vi "ml_K Means_Update Means.vi"(8 "# of classes":i32=1, 9 "labels":i32[](array[numeric]), 11 "Samples":dbl[][](array[numeric])) -> (0 "# samples in classes":i32[](array[numeric]), 1 "labels dup":i32[](array[numeric]), 2 "Means":dbl[][](array[numeric]), 3 "Samples dup":dbl[][](array[numeric]))   [LabVIEW 2013, in "NILabs_MLT.lvlib"]
uses:
  <vilib>/addons/Machine Learning/NILabs_MLT.lvlib
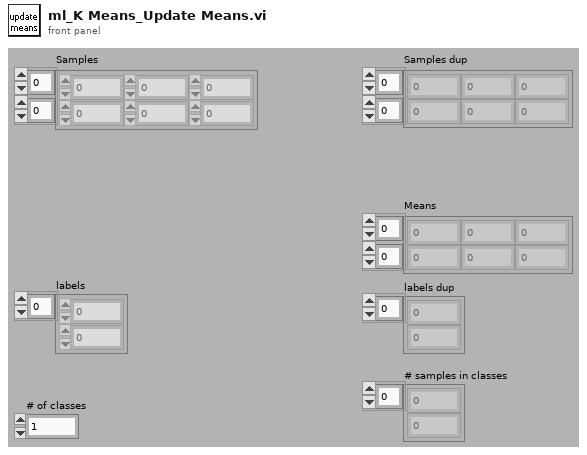
[diagram p1: front panel]
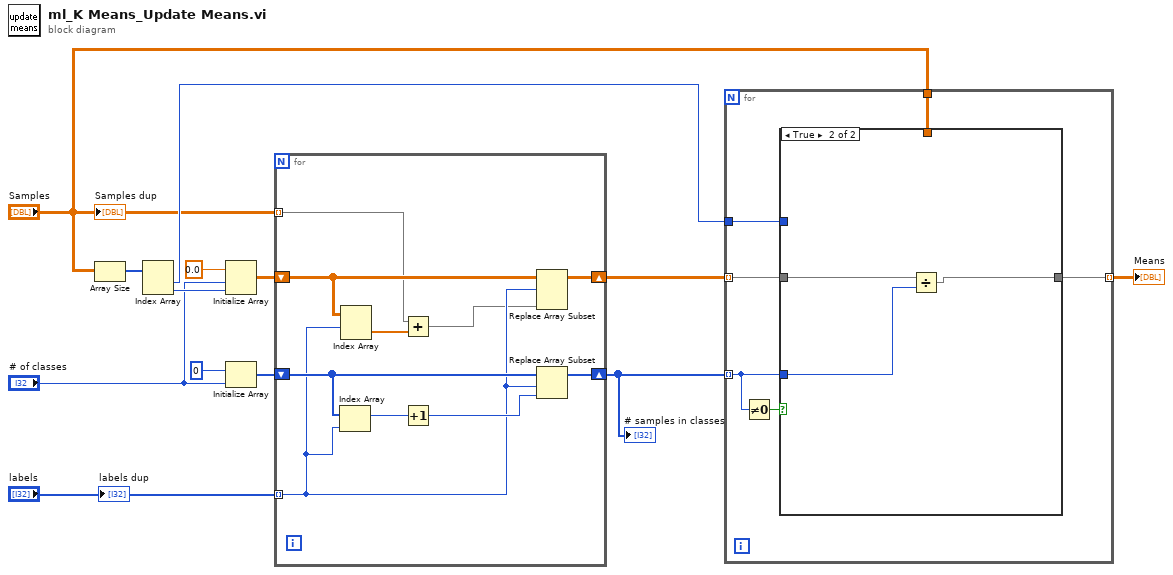
[diagram p0: block diagram]
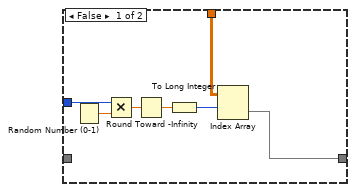
[diagram p2: hidden frame]
diagram:
  n1 = Array Size(array="Samples") -> (size(s)=w13:i32[])
  n2 = Index Array(array=w13) -> (element #1=w5:i32, element #2=w8:i32)  [unwired: 2 in]
  n3 = Initialize Array(0.0 ("element"), "# of classes", w8) -> (w9:dbl[][])
  n4 = Initialize Array(0 ("element"), "# of classes") -> (w10:i32[])
  n5 = for {
    tunnel: "labels" -> [w17] mode=indexing
    shift-right: [w19] -> w6
    shift-left: w9 -> [w20]
    shift-right: [w22] -> w2
    shift-left: w10 -> [w23]
    tunnel: "Samples" -> [w16] mode=indexing
    n6 = Index Array(array=w23, index=w17) -> (element=w18:i32)
    n7 = Index Array(array=w20, index (row)=w17) -> (element=w15:dbl[])  [unwired: 1 in]
    n8 = Add(x=w16, y=w15) -> (x+y=w14:dbl[])
    n9 = Increment(x=w18) -> (x+1=w21:i32)
    n10 = Replace Array Subset(array=w20, new element=w14, index (row)=w17) -> (w19:dbl[][])  [unwired: 1 in]
    n11 = Replace Array Subset(array=w23, new element=w21, index=w17) -> (w22:i32[])
  }
  "# samples in classes" <- w2
  n12 = for {
    tunnel: w6 -> [w28] mode=indexing
    tunnel: w2 -> [w27] mode=indexing
    tunnel: [w26] -> w3 mode=indexing
    tunnel: "Samples" -> [w25]
    tunnel: w5 -> [w24]
    n13 = Not Equal To 0?(x=w27) -> (x != 0?=w29:bool)
    n14 = case shown="True" w29 {
      tunnel: w28 -> [_ w39]
      tunnel: w27 -> [_ w38]
      tunnel: [w30 w37] -> w26
      tunnel: w25 -> [w32 _]
      tunnel: w24 -> [w35 _]
      frame False {
        n15 = Random Number (0-1)() -> (number: 0 to 1=w36:dbl)
        n16 = Multiply(x=w35, y=w36) -> (x*y=w34:dbl)
        n17 = Round Toward -Infinity(1:w34) -> (0:w33:dbl)
        n18 = To Long Integer(number=w33) -> (32bit integer=w31:i32)
        n19 = Index Array(array=w32, index (row)=w31) -> (element=w30:dbl[])  [unwired: 1 in]
      }
      frame True {
        n20 = Divide(x=w39, y=w38) -> (x/y=w37:dbl[])
      }
    }
  }
  "Means" <- w3
  "Samples dup" <- "Samples"
  "labels dup" <- "labels"
